vi "メイン.vi"() -> (2 "測定周期/ms":dbl, 3 "値転記用配列":T2[](array[typedef]))   [LabVIEW 2021] (continued)
        n4326 = for {
          N: w6937 -> [_]
          tunnel: FALSE -> [w6949]
          i -> [w6950]
          n4327 = case shown="5" w6950 {
            tunnel: w6949 -> [w6951 w6952 w6953 w6954 w6955 _ w6956 w6957 w6958 w6959 w6960 w6961]
            frame 0, Default {
              n4328 = local write "測定新値\nリセット用 1"(w6951) -> ()
            }
            frame 1 {
              n4329 = local write "測定新値\nリセット用 2"(w6952) -> ()
            }
            frame 2 {
              n4330 = local write "測定新値\nリセット用 3"(w6953) -> ()
            }
            frame 3 {
              n4331 = local write "測定新値\nリセット用 4"(w6954) -> ()
            }
            frame 4 {
              n4332 = local write "測定新値\nリセット用 5"(w6955) -> ()
            }
            frame 5 {
            }
            frame 6 {
              n4333 = local write "測定新値\nリセット用 7"(w6956) -> ()
            }
            frame 7 {
              n4334 = local write "測定新値\nリセット用 8"(w6957) -> ()
            }
            frame 8 {
              n4335 = local write "測定新値\nリセット用 9"(w6958) -> ()
            }
            frame 9 {
              n4336 = local write "測定新値\nリセット用 10"(w6959) -> ()
            }
            frame 10 {
              n4337 = local write "測定新値\nリセット用 11"(w6960) -> ()
            }
            frame 11 {
              n4338 = local write "測定新値\nリセット用 12"(w6961) -> ()
            }
          }
        }
        n4339 = for {
          N: w6937 -> [_]
          tunnel: w6943 -> [w6962]
          i -> [w6963]
          n4340 = case shown="11" w6963 {
            tunnel: w6962 -> [w6964 w6965 w6966 w6967 w6968 w6969 w6970 w6971 w6972 w6973 w6974 w6975]
            frame 0, Default {
              n4341 = property on="メイン測定ボタン_単発 1" class="Bool (指定)"("DisabledEnum"=w6964) -> ()  [unwired: 2 in, 2 out]
              n4342 = property on="メイン測定ボタン_連続 1" class="Bool (指定)"("DisabledEnum"=w6964) -> ()  [unwired: 2 in, 2 out]
            }
            frame 1 {
              n4343 = property on="メイン測定ボタン_単発 2" class="Bool (指定)"("DisabledEnum"=w6965) -> ()  [unwired: 2 in, 2 out]
              n4344 = property on="メイン測定ボタン_連続 2" class="Bool (指定)"("DisabledEnum"=w6965) -> ()  [unwired: 2 in, 2 out]
            }
            frame 2 {
              n4345 = property on="メイン測定ボタン_単発 3" class="Bool (指定)"("DisabledEnum"=w6966) -> ()  [unwired: 2 in, 2 out]
              n4346 = property on="メイン測定ボタン_連続 3" class="Bool (指定)"("DisabledEnum"=w6966) -> ()  [unwired: 2 in, 2 out]
            }
            frame 3 {
              n4347 = property on="メイン測定ボタン_単発 4" class="Bool (指定)"("DisabledEnum"=w6967) -> ()  [unwired: 2 in, 2 out]
              n4348 = property on="メイン測定ボタン_連続 4" class="Bool (指定)"("DisabledEnum"=w6967) -> ()  [unwired: 2 in, 2 out]
            }
            frame 4 {
              n4349 = property on="メイン測定ボタン_単発 5" class="Bool (指定)"("DisabledEnum"=w6968) -> ()  [unwired: 2 in, 2 out]
              n4350 = property on="メイン測定ボタン_連続 5" class="Bool (指定)"("DisabledEnum"=w6968) -> ()  [unwired: 2 in, 2 out]
            }
            frame 5 {
              n4351 = property on="メイン測定ボタン_単発 6" class="Bool (指定)"("DisabledEnum"=w6969) -> ()  [unwired: 2 in, 2 out]
            }
            frame 6 {
              n4352 = property on="メイン測定ボタン_連続 7" class="Bool (指定)"("DisabledEnum"=w6970) -> ()  [unwired: 2 in, 2 out]
              n4353 = property on="メイン測定ボタン_単発 7" class="Bool (指定)"("DisabledEnum"=w6970) -> ()  [unwired: 2 in, 2 out]
            }
            frame 7 {
              n4354 = property on="メイン測定ボタン_単発 8" class="Bool (指定)"("DisabledEnum"=w6971) -> ()  [unwired: 2 in, 2 out]
              n4355 = property on="メイン測定ボタン_連続 8" class="Bool (指定)"("DisabledEnum"=w6971) -> ()  [unwired: 2 in, 2 out]
            }
            frame 8 {
              n4356 = property on="メイン測定ボタン_単発 9" class="Bool (指定)"("DisabledEnum"=w6972) -> ()  [unwired: 2 in, 2 out]
              n4357 = property on="メイン測定ボタン_連続 9" class="Bool (指定)"("DisabledEnum"=w6972) -> ()  [unwired: 2 in, 2 out]
            }
            frame 9 {
              n4358 = property on="メイン測定ボタン_単発 10" class="Bool (指定)"("DisabledEnum"=w6973) -> ()  [unwired: 2 in, 2 out]
              n4359 = property on="メイン測定ボタン_連続 10" class="Bool (指定)"("DisabledEnum"=w6973) -> ()  [unwired: 2 in, 2 out]
            }
            frame 10 {
              n4360 = property on="メイン測定ボタン_単発 11" class="Bool (指定)"("DisabledEnum"=w6974) -> ()  [unwired: 2 in, 2 out]
              n4361 = property on="メイン測定ボタン_連続 11" class="Bool (指定)"("DisabledEnum"=w6974) -> ()  [unwired: 2 in, 2 out]
            }
            frame 11 {
              n4362 = property on="メイン測定ボタン_連続 12" class="Bool (指定)"("DisabledEnum"=w6975) -> ()  [unwired: 2 in, 2 out]
              n4363 = property on="メイン測定ボタン_単発 12" class="Bool (指定)"("DisabledEnum"=w6975) -> ()  [unwired: 2 in, 2 out]
            }
          }
        }
        n4364 = property on="TOPページへ" class="Bool"("DisabledEnum"=w6943) -> ()  [unwired: 2 in, 2 out]
        n4365 = property on="保存して終了" class="Bool"("DisabledEnum"=w6943) -> ()  [unwired: 2 in, 2 out]
        n4366 = property on="保存せずに" class="Bool"("DisabledEnum"=w6943) -> ()  [unwired: 2 in, 2 out]
      }
      event Value Change {
        w6976 = 12
        # "④ボタン操作時の他のボタン操作無効"
        # "※複製時\n①ブールボタン\n測定旧値\nが複製されているか確認\n②測定新値リセット用の作成\n対象の以外をリセットする\n③\nキュー\n④対象の連続ボタン以外複製する"
        # "③"
        # "旧値(ボタンが押される前と後)の値でグローバル_測定キャンセルボタンの\nTrue/Falseの切り替えを行う"
        # "②　例ケースが”メイン測定ボタン_連続2”の場合、\n測定新値リセット用2以外をリセットする"
        # "①"
        n4367 = event-data() -> ("OldVal"=w6978:T6)  [unwired: 1 in, 2 out]
        "測定旧値 7" <- w6978
        n4368 = Enqueue Element(queue=w6986, element="測定7", error in (no error)=w6983) -> (queue out=w6985:refnum<queue>, error out=w6984:errorcluster)  [unwired: 1 in, 1 out]
        n4369 = Select(t=TRUE, s=w6978, f=FALSE) -> (s? t:f=w6981:bool)
        n4370 = global write "測定キャンセルボタン.vi" "グローバル_測定キャンセルボタン"(w6981) -> ()
        n4371 = local write "G_メイン測定キャンセルボタン"(w6981) -> ()
        n4372 = for {
          N: w6976 -> [_]
          tunnel: FALSE -> [w6988]
          i -> [w6989]
          n4373 = case shown="6" w6989 {
            tunnel: w6988 -> [w6990 w6991 w6992 w6993 w6994 w6995 _ w6996 w6997 w6998 w6999 w7000]
            frame 0, Default {
              n4374 = local write "測定新値\nリセット用 1"(w6990) -> ()
            }
            frame 1 {
              n4375 = local write "測定新値\nリセット用 2"(w6991) -> ()
            }
            frame 2 {
              n4376 = local write "測定新値\nリセット用 3"(w6992) -> ()
            }
            frame 3 {
              n4377 = local write "測定新値\nリセット用 4"(w6993) -> ()
            }
            frame 4 {
              n4378 = local write "測定新値\nリセット用 5"(w6994) -> ()
            }
            frame 5 {
              n4379 = local write "測定新値\nリセット用 6"(w6995) -> ()
            }
            frame 6 {
            }
            frame 7 {
              n4380 = local write "測定新値\nリセット用 8"(w6996) -> ()
            }
            frame 8 {
              n4381 = local write "測定新値\nリセット用 9"(w6997) -> ()
            }
            frame 9 {
              n4382 = local write "測定新値\nリセット用 10"(w6998) -> ()
            }
            frame 10 {
              n4383 = local write "測定新値\nリセット用 11"(w6999) -> ()
            }
            frame 11 {
              n4384 = local write "測定新値\nリセット用 12"(w7000) -> ()
            }
          }
        }
        n4385 = for {
          N: w6976 -> [_]
          tunnel: w6982 -> [w7001]
          i -> [w7002]
          n4386 = case shown="11" w7002 {
            tunnel: w7001 -> [w7003 w7004 w7005 w7006 w7007 w7008 w7009 w7010 w7011 w7012 w7013 w7014]
            frame 0, Default {
              n4387 = property on="メイン測定ボタン_単発 1" class="Bool (指定)"("DisabledEnum"=w7003) -> ()  [unwired: 2 in, 2 out]
              n4388 = property on="メイン測定ボタン_連続 1" class="Bool (指定)"("DisabledEnum"=w7003) -> ()  [unwired: 2 in, 2 out]
            }
            frame 1 {
              n4389 = property on="メイン測定ボタン_単発 2" class="Bool (指定)"("DisabledEnum"=w7004) -> ()  [unwired: 2 in, 2 out]
              n4390 = property on="メイン測定ボタン_連続 2" class="Bool (指定)"("DisabledEnum"=w7004) -> ()  [unwired: 2 in, 2 out]
            }
            frame 2 {
              n4391 = property on="メイン測定ボタン_単発 3" class="Bool (指定)"("DisabledEnum"=w7005) -> ()  [unwired: 2 in, 2 out]
              n4392 = property on="メイン測定ボタン_連続 3" class="Bool (指定)"("DisabledEnum"=w7005) -> ()  [unwired: 2 in, 2 out]
            }
            frame 3 {
              n4393 = property on="メイン測定ボタン_単発 4" class="Bool (指定)"("DisabledEnum"=w7006) -> ()  [unwired: 2 in, 2 out]
              n4394 = property on="メイン測定ボタン_連続 4" class="Bool (指定)"("DisabledEnum"=w7006) -> ()  [unwired: 2 in, 2 out]
            }
            frame 4 {
              n4395 = property on="メイン測定ボタン_単発 5" class="Bool (指定)"("DisabledEnum"=w7007) -> ()  [unwired: 2 in, 2 out]
              n4396 = property on="メイン測定ボタン_連続 5" class="Bool (指定)"("DisabledEnum"=w7007) -> ()  [unwired: 2 in, 2 out]
            }
            frame 5 {
              n4397 = property on="メイン測定ボタン_連続 6" class="Bool (指定)"("DisabledEnum"=w7008) -> ()  [unwired: 2 in, 2 out]
              n4398 = property on="メイン測定ボタン_単発 6" class="Bool (指定)"("DisabledEnum"=w7008) -> ()  [unwired: 2 in, 2 out]
            }
            frame 6 {
              n4399 = property on="メイン測定ボタン_単発 7" class="Bool (指定)"("DisabledEnum"=w7009) -> ()  [unwired: 2 in, 2 out]
            }
            frame 7 {
              n4400 = property on="メイン測定ボタン_単発 8" class="Bool (指定)"("DisabledEnum"=w7010) -> ()  [unwired: 2 in, 2 out]
              n4401 = property on="メイン測定ボタン_連続 8" class="Bool (指定)"("DisabledEnum"=w7010) -> ()  [unwired: 2 in, 2 out]
            }
            frame 8 {
              n4402 = property on="メイン測定ボタン_単発 9" class="Bool (指定)"("DisabledEnum"=w7011) -> ()  [unwired: 2 in, 2 out]
              n4403 = property on="メイン測定ボタン_連続 9" class="Bool (指定)"("DisabledEnum"=w7011) -> ()  [unwired: 2 in, 2 out]
            }
            frame 9 {
              n4404 = property on="メイン測定ボタン_単発 10" class="Bool (指定)"("DisabledEnum"=w7012) -> ()  [unwired: 2 in, 2 out]
              n4405 = property on="メイン測定ボタン_連続 10" class="Bool (指定)"("DisabledEnum"=w7012) -> ()  [unwired: 2 in, 2 out]
            }
            frame 10 {
              n4406 = property on="メイン測定ボタン_単発 11" class="Bool (指定)"("DisabledEnum"=w7013) -> ()  [unwired: 2 in, 2 out]
              n4407 = property on="メイン測定ボタン_連続 11" class="Bool (指定)"("DisabledEnum"=w7013) -> ()  [unwired: 2 in, 2 out]
            }
            frame 11 {
              n4408 = property on="メイン測定ボタン_連続 12" class="Bool (指定)"("DisabledEnum"=w7014) -> ()  [unwired: 2 in, 2 out]
              n4409 = property on="メイン測定ボタン_単発 12" class="Bool (指定)"("DisabledEnum"=w7014) -> ()  [unwired: 2 in, 2 out]
            }
          }
        }
        n4410 = property on="TOPページへ" class="Bool"("DisabledEnum"=w6982) -> ()  [unwired: 2 in, 2 out]
        n4411 = property on="保存して終了" class="Bool"("DisabledEnum"=w6982) -> ()  [unwired: 2 in, 2 out]
        n4412 = property on="保存せずに" class="Bool"("DisabledEnum"=w6982) -> ()  [unwired: 2 in, 2 out]
      }
      event Value Change {
        w7015 = 12
        # "④ボタン操作時の他のボタン操作無効"
        # "※複製時\n①ブールボタン\n測定旧値\nが複製されているか確認\n②測定新値リセット用の作成\n対象の以外をリセットする\n③\nキュー\n④対象の連続ボタン以外複製する"
        # "③"
        # "旧値(ボタンが押される前と後)の値でグローバル_測定キャンセルボタンの\nTrue/Falseの切り替えを行う"
        # "②　例ケースが”メイン測定ボタン_連続2”の場合、\n測定新値リセット用2以外をリセットする"
        # "①"
        n4413 = event-data() -> ("OldVal"=w7017:T6)  [unwired: 1 in, 2 out]
        "測定旧値 8" <- w7017
        n4414 = Enqueue Element(queue=w7025, element="測定8", error in (no error)=w7022) -> (queue out=w7024:refnum<queue>, error out=w7023:errorcluster)  [unwired: 1 in, 1 out]
        n4415 = Select(t=TRUE, s=w7017, f=FALSE) -> (s? t:f=w7020:bool)
        n4416 = global write "測定キャンセルボタン.vi" "グローバル_測定キャンセルボタン"(w7020) -> ()
        n4417 = local write "G_メイン測定キャンセルボタン"(w7020) -> ()
        n4418 = for {
          N: w7015 -> [_]
          tunnel: FALSE -> [w7027]
          i -> [w7028]
          n4419 = case shown="7" w7028 {
            tunnel: w7027 -> [w7029 w7030 w7031 w7032 w7033 w7034 w7035 _ w7036 w7037 w7038 w7039]
            frame 0, Default {
              n4420 = local write "測定新値\nリセット用 1"(w7029) -> ()
            }
            frame 1 {
              n4421 = local write "測定新値\nリセット用 2"(w7030) -> ()
            }
            frame 2 {
              n4422 = local write "測定新値\nリセット用 3"(w7031) -> ()
            }
            frame 3 {
              n4423 = local write "測定新値\nリセット用 4"(w7032) -> ()
            }
            frame 4 {
              n4424 = local write "測定新値\nリセット用 5"(w7033) -> ()
            }
            frame 5 {
              n4425 = local write "測定新値\nリセット用 6"(w7034) -> ()
            }
            frame 6 {
              n4426 = local write "測定新値\nリセット用 7"(w7035) -> ()
            }
            frame 7 {
            }
            frame 8 {
              n4427 = local write "測定新値\nリセット用 9"(w7036) -> ()
            }
            frame 9 {
              n4428 = local write "測定新値\nリセット用 10"(w7037) -> ()
            }
            frame 10 {
              n4429 = local write "測定新値\nリセット用 11"(w7038) -> ()
            }
            frame 11 {
              n4430 = local write "測定新値\nリセット用 12"(w7039) -> ()
            }
          }
        }
        n4431 = for {
          N: w7015 -> [_]
          tunnel: w7021 -> [w7040]
          i -> [w7041]
          n4432 = case shown="11" w7041 {
            tunnel: w7040 -> [w7042 w7043 w7044 w7045 w7046 w7047 w7048 w7049 w7050 w7051 w7052 w7053]
            frame 0, Default {
              n4433 = property on="メイン測定ボタン_単発 1" class="Bool (指定)"("DisabledEnum"=w7042) -> ()  [unwired: 2 in, 2 out]
              n4434 = property on="メイン測定ボタン_連続 1" class="Bool (指定)"("DisabledEnum"=w7042) -> ()  [unwired: 2 in, 2 out]
            }
            frame 1 {
              n4435 = property on="メイン測定ボタン_単発 2" class="Bool (指定)"("DisabledEnum"=w7043) -> ()  [unwired: 2 in, 2 out]
              n4436 = property on="メイン測定ボタン_連続 2" class="Bool (指定)"("DisabledEnum"=w7043) -> ()  [unwired: 2 in, 2 out]
            }
            frame 2 {
              n4437 = property on="メイン測定ボタン_単発 3" class="Bool (指定)"("DisabledEnum"=w7044) -> ()  [unwired: 2 in, 2 out]
              n4438 = property on="メイン測定ボタン_連続 3" class="Bool (指定)"("DisabledEnum"=w7044) -> ()  [unwired: 2 in, 2 out]
            }
            frame 3 {
              n4439 = property on="メイン測定ボタン_単発 4" class="Bool (指定)"("DisabledEnum"=w7045) -> ()  [unwired: 2 in, 2 out]
              n4440 = property on="メイン測定ボタン_連続 4" class="Bool (指定)"("DisabledEnum"=w7045) -> ()  [unwired: 2 in, 2 out]
            }
            frame 4 {
              n4441 = property on="メイン測定ボタン_単発 5" class="Bool (指定)"("DisabledEnum"=w7046) -> ()  [unwired: 2 in, 2 out]
              n4442 = property on="メイン測定ボタン_連続 5" class="Bool (指定)"("DisabledEnum"=w7046) -> ()  [unwired: 2 in, 2 out]
            }
            frame 5 {
              n4443 = property on="メイン測定ボタン_連続 6" class="Bool (指定)"("DisabledEnum"=w7047) -> ()  [unwired: 2 in, 2 out]
              n4444 = property on="メイン測定ボタン_単発 6" class="Bool (指定)"("DisabledEnum"=w7047) -> ()  [unwired: 2 in, 2 out]
            }
            frame 6 {
              n4445 = property on="メイン測定ボタン_連続 7" class="Bool (指定)"("DisabledEnum"=w7048) -> ()  [unwired: 2 in, 2 out]
              n4446 = property on="メイン測定ボタン_単発 7" class="Bool (指定)"("DisabledEnum"=w7048) -> ()  [unwired: 2 in, 2 out]
            }
            frame 7 {
              n4447 = property on="メイン測定ボタン_単発 8" class="Bool (指定)"("DisabledEnum"=w7049) -> ()  [unwired: 2 in, 2 out]
            }
            frame 8 {
              n4448 = property on="メイン測定ボタン_単発 9" class="Bool (指定)"("DisabledEnum"=w7050) -> ()  [unwired: 2 in, 2 out]
              n4449 = property on="メイン測定ボタン_連続 9" class="Bool (指定)"("DisabledEnum"=w7050) -> ()  [unwired: 2 in, 2 out]
            }
            frame 9 {
              n4450 = property on="メイン測定ボタン_単発 10" class="Bool (指定)"("DisabledEnum"=w7051) -> ()  [unwired: 2 in, 2 out]
              n4451 = property on="メイン測定ボタン_連続 10" class="Bool (指定)"("DisabledEnum"=w7051) -> ()  [unwired: 2 in, 2 out]
            }
            frame 10 {
              n4452 = property on="メイン測定ボタン_単発 11" class="Bool (指定)"("DisabledEnum"=w7052) -> ()  [unwired: 2 in, 2 out]
              n4453 = property on="メイン測定ボタン_連続 11" class="Bool (指定)"("DisabledEnum"=w7052) -> ()  [unwired: 2 in, 2 out]
            }
            frame 11 {
              n4454 = property on="メイン測定ボタン_連続 12" class="Bool (指定)"("DisabledEnum"=w7053) -> ()  [unwired: 2 in, 2 out]
              n4455 = property on="メイン測定ボタン_単発 12" class="Bool (指定)"("DisabledEnum"=w7053) -> ()  [unwired: 2 in, 2 out]
            }
          }
        }
        n4456 = property on="TOPページへ" class="Bool"("DisabledEnum"=w7021) -> ()  [unwired: 2 in, 2 out]
        n4457 = property on="保存して終了" class="Bool"("DisabledEnum"=w7021) -> ()  [unwired: 2 in, 2 out]
        n4458 = property on="保存せずに" class="Bool"("DisabledEnum"=w7021) -> ()  [unwired: 2 in, 2 out]
      }
      event Value Change {
        w7054 = 12
        # "④ボタン操作時の他のボタン操作無効"
        # "※複製時\n①ブールボタン\n測定旧値\nが複製されているか確認\n②測定新値リセット用の作成\n対象の以外をリセットする\n③\nキュー\n④対象の連続ボタン以外複製する"
        # "③"
        # "旧値(ボタンが押される前と後)の値でグローバル_測定キャンセルボタンの\nTrue/Falseの切り替えを行う"
        # "②　例ケースが”メイン測定ボタン_連続2”の場合、\n測定新値リセット用2以外をリセットする"
        # "①"
        n4459 = event-data() -> ("OldVal"=w7056:T6)  [unwired: 1 in, 2 out]
        "測定旧値 9" <- w7056
        n4460 = Enqueue Element(queue=w7064, element="測定9", error in (no error)=w7061) -> (queue out=w7063:refnum<queue>, error out=w7062:errorcluster)  [unwired: 1 in, 1 out]
        n4461 = Select(t=TRUE, s=w7056, f=FALSE) -> (s? t:f=w7059:bool)
        n4462 = global write "測定キャンセルボタン.vi" "グローバル_測定キャンセルボタン"(w7059) -> ()
        n4463 = local write "G_メイン測定キャンセルボタン"(w7059) -> ()
        n4464 = for {
          N: w7054 -> [_]
          tunnel: FALSE -> [w7066]
          i -> [w7067]
          n4465 = case shown="8" w7067 {
            tunnel: w7066 -> [w7068 w7069 w7070 w7071 w7072 w7073 w7074 w7075 _ w7076 w7077 w7078]
            frame 0, Default {
              n4466 = local write "測定新値\nリセット用 1"(w7068) -> ()
            }
            frame 1 {
              n4467 = local write "測定新値\nリセット用 2"(w7069) -> ()
            }
            frame 2 {
              n4468 = local write "測定新値\nリセット用 3"(w7070) -> ()
            }
            frame 3 {
              n4469 = local write "測定新値\nリセット用 4"(w7071) -> ()
            }
            frame 4 {
              n4470 = local write "測定新値\nリセット用 5"(w7072) -> ()
            }
            frame 5 {
              n4471 = local write "測定新値\nリセット用 6"(w7073) -> ()
            }
            frame 6 {
              n4472 = local write "測定新値\nリセット用 7"(w7074) -> ()
            }
            frame 7 {
              n4473 = local write "測定新値\nリセット用 8"(w7075) -> ()
            }
            frame 8 {
            }
            frame 9 {
              n4474 = local write "測定新値\nリセット用 10"(w7076) -> ()
            }
            frame 10 {
              n4475 = local write "測定新値\nリセット用 11"(w7077) -> ()
            }
            frame 11 {
              n4476 = local write "測定新値\nリセット用 12"(w7078) -> ()
            }
          }
        }
        n4477 = for {
          N: w7054 -> [_]
          tunnel: w7060 -> [w7079]
          i -> [w7080]
          n4478 = case shown="11" w7080 {
            tunnel: w7079 -> [w7081 w7082 w7083 w7084 w7085 w7086 w7087 w7088 w7089 w7090 w7091 w7092]
            frame 0, Default {
              n4479 = property on="メイン測定ボタン_単発 1" class="Bool (指定)"("DisabledEnum"=w7081) -> ()  [unwired: 2 in, 2 out]
              n4480 = property on="メイン測定ボタン_連続 1" class="Bool (指定)"("DisabledEnum"=w7081) -> ()  [unwired: 2 in, 2 out]
            }
            frame 1 {
              n4481 = property on="メイン測定ボタン_単発 2" class="Bool (指定)"("DisabledEnum"=w7082) -> ()  [unwired: 2 in, 2 out]
              n4482 = property on="メイン測定ボタン_連続 2" class="Bool (指定)"("DisabledEnum"=w7082) -> ()  [unwired: 2 in, 2 out]
            }
            frame 2 {
              n4483 = property on="メイン測定ボタン_単発 3" class="Bool (指定)"("DisabledEnum"=w7083) -> ()  [unwired: 2 in, 2 out]
              n4484 = property on="メイン測定ボタン_連続 3" class="Bool (指定)"("DisabledEnum"=w7083) -> ()  [unwired: 2 in, 2 out]
            }
            frame 3 {
              n4485 = property on="メイン測定ボタン_単発 4" class="Bool (指定)"("DisabledEnum"=w7084) -> ()  [unwired: 2 in, 2 out]
              n4486 = property on="メイン測定ボタン_連続 4" class="Bool (指定)"("DisabledEnum"=w7084) -> ()  [unwired: 2 in, 2 out]
            }
            frame 4 {
              n4487 = property on="メイン測定ボタン_単発 5" class="Bool (指定)"("DisabledEnum"=w7085) -> ()  [unwired: 2 in, 2 out]
              n4488 = property on="メイン測定ボタン_連続 5" class="Bool (指定)"("DisabledEnum"=w7085) -> ()  [unwired: 2 in, 2 out]
            }
            frame 5 {
              n4489 = property on="メイン測定ボタン_連続 6" class="Bool (指定)"("DisabledEnum"=w7086) -> ()  [unwired: 2 in, 2 out]
              n4490 = property on="メイン測定ボタン_単発 6" class="Bool (指定)"("DisabledEnum"=w7086) -> ()  [unwired: 2 in, 2 out]
            }
            frame 6 {
              n4491 = property on="メイン測定ボタン_連続 7" class="Bool (指定)"("DisabledEnum"=w7087) -> ()  [unwired: 2 in, 2 out]
              n4492 = property on="メイン測定ボタン_単発 7" class="Bool (指定)"("DisabledEnum"=w7087) -> ()  [unwired: 2 in, 2 out]
            }
            frame 7 {
              n4493 = property on="メイン測定ボタン_単発 8" class="Bool (指定)"("DisabledEnum"=w7088) -> ()  [unwired: 2 in, 2 out]
              n4494 = property on="メイン測定ボタン_連続 8" class="Bool (指定)"("DisabledEnum"=w7088) -> ()  [unwired: 2 in, 2 out]
            }
            frame 8 {
              n4495 = property on="メイン測定ボタン_単発 9" class="Bool (指定)"("DisabledEnum"=w7089) -> ()  [unwired: 2 in, 2 out]
            }
            frame 9 {
              n4496 = property on="メイン測定ボタン_単発 10" class="Bool (指定)"("DisabledEnum"=w7090) -> ()  [unwired: 2 in, 2 out]
              n4497 = property on="メイン測定ボタン_連続 10" class="Bool (指定)"("DisabledEnum"=w7090) -> ()  [unwired: 2 in, 2 out]
            }
            frame 10 {
              n4498 = property on="メイン測定ボタン_単発 11" class="Bool (指定)"("DisabledEnum"=w7091) -> ()  [unwired: 2 in, 2 out]
              n4499 = property on="メイン測定ボタン_連続 11" class="Bool (指定)"("DisabledEnum"=w7091) -> ()  [unwired: 2 in, 2 out]
            }
            frame 11 {
              n4500 = property on="メイン測定ボタン_連続 12" class="Bool (指定)"("DisabledEnum"=w7092) -> ()  [unwired: 2 in, 2 out]
              n4501 = property on="メイン測定ボタン_単発 12" class="Bool (指定)"("DisabledEnum"=w7092) -> ()  [unwired: 2 in, 2 out]
            }
          }
        }
        n4502 = property on="TOPページへ" class="Bool"("DisabledEnum"=w7060) -> ()  [unwired: 2 in, 2 out]
        n4503 = property on="保存して終了" class="Bool"("DisabledEnum"=w7060) -> ()  [unwired: 2 in, 2 out]
        n4504 = property on="保存せずに" class="Bool"("DisabledEnum"=w7060) -> ()  [unwired: 2 in, 2 out]
      }
      event Value Change {
        w7093 = 12
        # "④ボタン操作時の他のボタン操作無効"
        # "※複製時\n①ブールボタン\n測定旧値\nが複製されているか確認\n②測定新値リセット用の作成\n対象の以外をリセットする\n③\nキュー\n④対象の連続ボタン以外複製する"
        # "③"
        # "旧値(ボタンが押される前と後)の値でグローバル_測定キャンセルボタンの\nTrue/Falseの切り替えを行う"
        # "②　例ケースが”メイン測定ボタン_連続2”の場合、\n測定新値リセット用2以外をリセットする"
        # "①"
        n4505 = event-data() -> ("OldVal"=w7095:T6)  [unwired: 1 in, 2 out]
        "測定旧値 10" <- w7095
        n4506 = Enqueue Element(queue=w7103, element="測定10", error in (no error)=w7100) -> (queue out=w7102:refnum<queue>, error out=w7101:errorcluster)  [unwired: 1 in, 1 out]
        n4507 = Select(t=TRUE, s=w7095, f=FALSE) -> (s? t:f=w7098:bool)
        n4508 = global write "測定キャンセルボタン.vi" "グローバル_測定キャンセルボタン"(w7098) -> ()
        n4509 = local write "G_メイン測定キャンセルボタン"(w7098) -> ()
        n4510 = for {
          N: w7093 -> [_]
          tunnel: FALSE -> [w7105]
          i -> [w7106]
          n4511 = case shown="9" w7106 {
            tunnel: w7105 -> [w7107 w7108 w7109 w7110 w7111 w7112 w7113 w7114 w7115 _ w7116 w7117]
            frame 0, Default {
              n4512 = local write "測定新値\nリセット用 1"(w7107) -> ()
            }
            frame 1 {
              n4513 = local write "測定新値\nリセット用 2"(w7108) -> ()
            }
            frame 2 {
              n4514 = local write "測定新値\nリセット用 3"(w7109) -> ()
            }
            frame 3 {
              n4515 = local write "測定新値\nリセット用 4"(w7110) -> ()
            }
            frame 4 {
              n4516 = local write "測定新値\nリセット用 5"(w7111) -> ()
            }
            frame 5 {
              n4517 = local write "測定新値\nリセット用 6"(w7112) -> ()
            }
            frame 6 {
              n4518 = local write "測定新値\nリセット用 7"(w7113) -> ()
            }
            frame 7 {
              n4519 = local write "測定新値\nリセット用 8"(w7114) -> ()
            }
            frame 8 {
              n4520 = local write "測定新値\nリセット用 9"(w7115) -> ()
            }
            frame 9 {
            }
            frame 10 {
              n4521 = local write "測定新値\nリセット用 11"(w7116) -> ()
            }
            frame 11 {
              n4522 = local write "測定新値\nリセット用 12"(w7117) -> ()
            }
          }
        }
        n4523 = for {
          N: w7093 -> [_]
          tunnel: w7099 -> [w7118]
          i -> [w7119]
          n4524 = case shown="11" w7119 {
            tunnel: w7118 -> [w7120 w7121 w7122 w7123 w7124 w7125 w7126 w7127 w7128 w7129 w7130 w7131]
            frame 0, Default {
              n4525 = property on="メイン測定ボタン_単発 1" class="Bool (指定)"("DisabledEnum"=w7120) -> ()  [unwired: 2 in, 2 out]
              n4526 = property on="メイン測定ボタン_連続 1" class="Bool (指定)"("DisabledEnum"=w7120) -> ()  [unwired: 2 in, 2 out]
            }
            frame 1 {
              n4527 = property on="メイン測定ボタン_単発 2" class="Bool (指定)"("DisabledEnum"=w7121) -> ()  [unwired: 2 in, 2 out]
              n4528 = property on="メイン測定ボタン_連続 2" class="Bool (指定)"("DisabledEnum"=w7121) -> ()  [unwired: 2 in, 2 out]
            }
            frame 2 {
              n4529 = property on="メイン測定ボタン_単発 3" class="Bool (指定)"("DisabledEnum"=w7122) -> ()  [unwired: 2 in, 2 out]
              n4530 = property on="メイン測定ボタン_連続 3" class="Bool (指定)"("DisabledEnum"=w7122) -> ()  [unwired: 2 in, 2 out]
            }
            frame 3 {
              n4531 = property on="メイン測定ボタン_単発 4" class="Bool (指定)"("DisabledEnum"=w7123) -> ()  [unwired: 2 in, 2 out]
              n4532 = property on="メイン測定ボタン_連続 4" class="Bool (指定)"("DisabledEnum"=w7123) -> ()  [unwired: 2 in, 2 out]
            }
            frame 4 {
              n4533 = property on="メイン測定ボタン_単発 5" class="Bool (指定)"("DisabledEnum"=w7124) -> ()  [unwired: 2 in, 2 out]
              n4534 = property on="メイン測定ボタン_連続 5" class="Bool (指定)"("DisabledEnum"=w7124) -> ()  [unwired: 2 in, 2 out]
            }
            frame 5 {
              n4535 = property on="メイン測定ボタン_連続 6" class="Bool (指定)"("DisabledEnum"=w7125) -> ()  [unwired: 2 in, 2 out]
              n4536 = property on="メイン測定ボタン_単発 6" class="Bool (指定)"("DisabledEnum"=w7125) -> ()  [unwired: 2 in, 2 out]
            }
            frame 6 {
              n4537 = property on="メイン測定ボタン_連続 7" class="Bool (指定)"("DisabledEnum"=w7126) -> ()  [unwired: 2 in, 2 out]
              n4538 = property on="メイン測定ボタン_単発 7" class="Bool (指定)"("DisabledEnum"=w7126) -> ()  [unwired: 2 in, 2 out]
            }
            frame 7 {
              n4539 = property on="メイン測定ボタン_単発 8" class="Bool (指定)"("DisabledEnum"=w7127) -> ()  [unwired: 2 in, 2 out]
              n4540 = property on="メイン測定ボタン_連続 8" class="Bool (指定)"("DisabledEnum"=w7127) -> ()  [unwired: 2 in, 2 out]
            }
            frame 8 {
              n4541 = property on="メイン測定ボタン_単発 9" class="Bool (指定)"("DisabledEnum"=w7128) -> ()  [unwired: 2 in, 2 out]
              n4542 = property on="メイン測定ボタン_連続 9" class="Bool (指定)"("DisabledEnum"=w7128) -> ()  [unwired: 2 in, 2 out]
            }
            frame 9 {
              n4543 = property on="メイン測定ボタン_単発 10" class="Bool (指定)"("DisabledEnum"=w7129) -> ()  [unwired: 2 in, 2 out]
            }
            frame 10 {
              n4544 = property on="メイン測定ボタン_単発 11" class="Bool (指定)"("DisabledEnum"=w7130) -> ()  [unwired: 2 in, 2 out]
              n4545 = property on="メイン測定ボタン_連続 11" class="Bool (指定)"("DisabledEnum"=w7130) -> ()  [unwired: 2 in, 2 out]
            }
            frame 11 {
              n4546 = property on="メイン測定ボタン_連続 12" class="Bool (指定)"("DisabledEnum"=w7131) -> ()  [unwired: 2 in, 2 out]
              n4547 = property on="メイン測定ボタン_単発 12" class="Bool (指定)"("DisabledEnum"=w7131) -> ()  [unwired: 2 in, 2 out]
            }
          }
        }
        n4548 = property on="TOPページへ" class="Bool"("DisabledEnum"=w7099) -> ()  [unwired: 2 in, 2 out]
        n4549 = property on="保存して終了" class="Bool"("DisabledEnum"=w7099) -> ()  [unwired: 2 in, 2 out]
        n4550 = property on="保存せずに" class="Bool"("DisabledEnum"=w7099) -> ()  [unwired: 2 in, 2 out]
      }
      event Value Change {
        w7132 = 12
        # "④ボタン操作時の他のボタン操作無効"
        # "※複製時\n①ブールボタン\n測定旧値\nが複製されているか確認\n②測定新値リセット用の作成\n対象の以外をリセットする\n③\nキュー\n④対象の連続ボタン以外複製する"
        # "③"
        # "旧値(ボタンが押される前と後)の値でグローバル_測定キャンセルボタンの\nTrue/Falseの切り替えを行う"
        # "②　例ケースが”メイン測定ボタン_連続2”の場合、\n測定新値リセット用2以外をリセットする"
        # "①"
        n4551 = event-data() -> ("OldVal"=w7134:T6)  [unwired: 1 in, 2 out]
        "測定旧値 11" <- w7134
        n4552 = Enqueue Element(queue=w7142, element="測定11", error in (no error)=w7139) -> (queue out=w7141:refnum<queue>, error out=w7140:errorcluster)  [unwired: 1 in, 1 out]
        n4553 = Select(t=TRUE, s=w7134, f=FALSE) -> (s? t:f=w7137:bool)
        n4554 = global write "測定キャンセルボタン.vi" "グローバル_測定キャンセルボタン"(w7137) -> ()
        n4555 = local write "G_メイン測定キャンセルボタン"(w7137) -> ()
        n4556 = for {
          N: w7132 -> [_]
          tunnel: FALSE -> [w7144]
          i -> [w7145]
          n4557 = case shown="10" w7145 {
            tunnel: w7144 -> [w7146 w7147 w7148 w7149 w7150 w7151 w7152 w7153 w7154 w7155 _ w7156]
            frame 0, Default {
              n4558 = local write "測定新値\nリセット用 1"(w7146) -> ()
            }
            frame 1 {
              n4559 = local write "測定新値\nリセット用 2"(w7147) -> ()
            }
            frame 2 {
              n4560 = local write "測定新値\nリセット用 3"(w7148) -> ()
            }
            frame 3 {
              n4561 = local write "測定新値\nリセット用 4"(w7149) -> ()
            }
            frame 4 {
              n4562 = local write "測定新値\nリセット用 5"(w7150) -> ()
            }
            frame 5 {
              n4563 = local write "測定新値\nリセット用 6"(w7151) -> ()
            }
            frame 6 {
              n4564 = local write "測定新値\nリセット用 7"(w7152) -> ()
            }
            frame 7 {
              n4565 = local write "測定新値\nリセット用 8"(w7153) -> ()
            }
            frame 8 {
              n4566 = local write "測定新値\nリセット用 9"(w7154) -> ()
            }
            frame 9 {
              n4567 = local write "測定新値\nリセット用 10"(w7155) -> ()
            }
            frame 10 {
            }
            frame 11 {
              n4568 = local write "測定新値\nリセット用 12"(w7156) -> ()
            }
          }
        }
        n4569 = for {
          N: w7132 -> [_]
          tunnel: w7138 -> [w7157]
          i -> [w7158]
          n4570 = case shown="11" w7158 {
            tunnel: w7157 -> [w7159 w7160 w7161 w7162 w7163 w7164 w7165 w7166 w7167 w7168 w7169 w7170]
            frame 0, Default {
              n4571 = property on="メイン測定ボタン_単発 1" class="Bool (指定)"("DisabledEnum"=w7159) -> ()  [unwired: 2 in, 2 out]
              n4572 = property on="メイン測定ボタン_連続 1" class="Bool (指定)"("DisabledEnum"=w7159) -> ()  [unwired: 2 in, 2 out]
            }
            frame 1 {
              n4573 = property on="メイン測定ボタン_単発 2" class="Bool (指定)"("DisabledEnum"=w7160) -> ()  [unwired: 2 in, 2 out]
              n4574 = property on="メイン測定ボタン_連続 2" class="Bool (指定)"("DisabledEnum"=w7160) -> ()  [unwired: 2 in, 2 out]
            }
            frame 2 {
              n4575 = property on="メイン測定ボタン_単発 3" class="Bool (指定)"("DisabledEnum"=w7161) -> ()  [unwired: 2 in, 2 out]
              n4576 = property on="メイン測定ボタン_連続 3" class="Bool (指定)"("DisabledEnum"=w7161) -> ()  [unwired: 2 in, 2 out]
            }
            frame 3 {
              n4577 = property on="メイン測定ボタン_単発 4" class="Bool (指定)"("DisabledEnum"=w7162) -> ()  [unwired: 2 in, 2 out]
              n4578 = property on="メイン測定ボタン_連続 4" class="Bool (指定)"("DisabledEnum"=w7162) -> ()  [unwired: 2 in, 2 out]
            }
            frame 4 {
              n4579 = property on="メイン測定ボタン_単発 5" class="Bool (指定)"("DisabledEnum"=w7163) -> ()  [unwired: 2 in, 2 out]
              n4580 = property on="メイン測定ボタン_連続 5" class="Bool (指定)"("DisabledEnum"=w7163) -> ()  [unwired: 2 in, 2 out]
            }
            frame 5 {
              n4581 = property on="メイン測定ボタン_連続 6" class="Bool (指定)"("DisabledEnum"=w7164) -> ()  [unwired: 2 in, 2 out]
              n4582 = property on="メイン測定ボタン_単発 6" class="Bool (指定)"("DisabledEnum"=w7164) -> ()  [unwired: 2 in, 2 out]
            }
            frame 6 {
              n4583 = property on="メイン測定ボタン_連続 7" class="Bool (指定)"("DisabledEnum"=w7165) -> ()  [unwired: 2 in, 2 out]
              n4584 = property on="メイン測定ボタン_単発 7" class="Bool (指定)"("DisabledEnum"=w7165) -> ()  [unwired: 2 in, 2 out]
            }
            frame 7 {
              n4585 = property on="メイン測定ボタン_単発 8" class="Bool (指定)"("DisabledEnum"=w7166) -> ()  [unwired: 2 in, 2 out]
              n4586 = property on="メイン測定ボタン_連続 8" class="Bool (指定)"("DisabledEnum"=w7166) -> ()  [unwired: 2 in, 2 out]
            }
            frame 8 {
              n4587 = property on="メイン測定ボタン_単発 9" class="Bool (指定)"("DisabledEnum"=w7167) -> ()  [unwired: 2 in, 2 out]
              n4588 = property on="メイン測定ボタン_連続 9" class="Bool (指定)"("DisabledEnum"=w7167) -> ()  [unwired: 2 in, 2 out]
            }
            frame 9 {
              n4589 = property on="メイン測定ボタン_単発 10" class="Bool (指定)"("DisabledEnum"=w7168) -> ()  [unwired: 2 in, 2 out]
              n4590 = property on="メイン測定ボタン_連続 10" class="Bool (指定)"("DisabledEnum"=w7168) -> ()  [unwired: 2 in, 2 out]
            }
            frame 10 {
              n4591 = property on="メイン測定ボタン_単発 11" class="Bool (指定)"("DisabledEnum"=w7169) -> ()  [unwired: 2 in, 2 out]
            }
            frame 11 {
              n4592 = property on="メイン測定ボタン_連続 12" class="Bool (指定)"("DisabledEnum"=w7170) -> ()  [unwired: 2 in, 2 out]
              n4593 = property on="メイン測定ボタン_単発 12" class="Bool (指定)"("DisabledEnum"=w7170) -> ()  [unwired: 2 in, 2 out]
            }
          }
        }
        n4594 = property on="TOPページへ" class="Bool"("DisabledEnum"=w7138) -> ()  [unwired: 2 in, 2 out]
        n4595 = property on="保存して終了" class="Bool"("DisabledEnum"=w7138) -> ()  [unwired: 2 in, 2 out]
        n4596 = property on="保存せずに" class="Bool"("DisabledEnum"=w7138) -> ()  [unwired: 2 in, 2 out]
      }
      event Value Change {
        w7171 = 12
        # "④ボタン操作時の他のボタン操作無効"
        # "※複製時\n①ブールボタン\n測定旧値\nが複製されているか確認\n②測定新値リセット用の作成\n対象の以外をリセットする\n③\nキュー\n④対象の連続ボタン以外複製する"
        # "③"
        # "旧値(ボタンが押される前と後)の値でグローバル_測定キャンセルボタンの\nTrue/Falseの切り替えを行う"
        # "②　例ケースが”メイン測定ボタン_連続2”の場合、\n測定新値リセット用2以外をリセットする"
        # "①"
        n4597 = event-data() -> ("OldVal"=w7172:T6)  [unwired: 1 in, 2 out]
        "測定旧値 12" <- w7172
        n4598 = Enqueue Element(queue=w7181, element="測定12", error in (no error)=w7178) -> (queue out=w7180:refnum<queue>, error out=w7179:errorcluster)  [unwired: 1 in, 1 out]
        n4599 = Select(t=TRUE, s=w7172, f=FALSE) -> (s? t:f=w7175:bool)
        n4600 = global write "測定キャンセルボタン.vi" "グローバル_測定キャンセルボタン"(w7175) -> ()
        n4601 = local write "G_メイン測定キャンセルボタン"(w7175) -> ()
        n4602 = for {
          N: w7171 -> [_]
          tunnel: FALSE -> [w7197]
          i -> [w7198]
          n4603 = case shown="0, デフォルト" w7198 {
            tunnel: w7197 -> [w7199 w7200 w7201 w7202 w7203 w7204 w7205 w7206 w7207 w7208 w7209]
            frame 0, Default {
              n4604 = local write "測定新値\nリセット用 1"(w7199) -> ()
            }
            frame 1 {
              n4605 = local write "測定新値\nリセット用 2"(w7200) -> ()
            }
            frame 2 {
              n4606 = local write "測定新値\nリセット用 3"(w7201) -> ()
            }
            frame 3 {
              n4607 = local write "測定新値\nリセット用 4"(w7202) -> ()
            }
            frame 4 {
              n4608 = local write "測定新値\nリセット用 5"(w7203) -> ()
            }
            frame 5 {
              n4609 = local write "測定新値\nリセット用 6"(w7204) -> ()
            }
            frame 6 {
              n4610 = local write "測定新値\nリセット用 7"(w7205) -> ()
            }
            frame 7 {
              n4611 = local write "測定新値\nリセット用 8"(w7206) -> ()
            }
            frame 8 {
              n4612 = local write "測定新値\nリセット用 9"(w7207) -> ()
            }
            frame 9 {
              n4613 = local write "測定新値\nリセット用 10"(w7208) -> ()
            }
            frame 10 {
              n4614 = local write "測定新値\nリセット用 11"(w7209) -> ()
            }
          }
        }
        n4615 = for {
          N: w7171 -> [_]
          tunnel: w7176 -> [w7183]
          i -> [w7184]
          n4616 = case shown="11" w7184 {
            tunnel: w7183 -> [w7185 w7186 w7187 w7188 w7189 w7190 w7191 w7192 w7193 w7194 w7195 w7196]
            frame 0, Default {
              n4617 = property on="メイン測定ボタン_単発 1" class="Bool (指定)"("DisabledEnum"=w7185) -> ()  [unwired: 2 in, 2 out]
              n4618 = property on="メイン測定ボタン_連続 1" class="Bool (指定)"("DisabledEnum"=w7185) -> ()  [unwired: 2 in, 2 out]
            }
            frame 1 {
              n4619 = property on="メイン測定ボタン_単発 2" class="Bool (指定)"("DisabledEnum"=w7186) -> ()  [unwired: 2 in, 2 out]
              n4620 = property on="メイン測定ボタン_連続 2" class="Bool (指定)"("DisabledEnum"=w7186) -> ()  [unwired: 2 in, 2 out]
            }
            frame 2 {
              n4621 = property on="メイン測定ボタン_単発 3" class="Bool (指定)"("DisabledEnum"=w7187) -> ()  [unwired: 2 in, 2 out]
              n4622 = property on="メイン測定ボタン_連続 3" class="Bool (指定)"("DisabledEnum"=w7187) -> ()  [unwired: 2 in, 2 out]
            }
            frame 3 {
              n4623 = property on="メイン測定ボタン_単発 4" class="Bool (指定)"("DisabledEnum"=w7188) -> ()  [unwired: 2 in, 2 out]
              n4624 = property on="メイン測定ボタン_連続 4" class="Bool (指定)"("DisabledEnum"=w7188) -> ()  [unwired: 2 in, 2 out]
            }
            frame 4 {
              n4625 = property on="メイン測定ボタン_単発 5" class="Bool (指定)"("DisabledEnum"=w7189) -> ()  [unwired: 2 in, 2 out]
              n4626 = property on="メイン測定ボタン_連続 5" class="Bool (指定)"("DisabledEnum"=w7189) -> ()  [unwired: 2 in, 2 out]
            }
            frame 5 {
              n4627 = property on="メイン測定ボタン_連続 6" class="Bool (指定)"("DisabledEnum"=w7190) -> ()  [unwired: 2 in, 2 out]
              n4628 = property on="メイン測定ボタン_単発 6" class="Bool (指定)"("DisabledEnum"=w7190) -> ()  [unwired: 2 in, 2 out]
            }
            frame 6 {
              n4629 = property on="メイン測定ボタン_連続 7" class="Bool (指定)"("DisabledEnum"=w7191) -> ()  [unwired: 2 in, 2 out]
              n4630 = property on="メイン測定ボタン_単発 7" class="Bool (指定)"("DisabledEnum"=w7191) -> ()  [unwired: 2 in, 2 out]
            }
            frame 7 {
              n4631 = property on="メイン測定ボタン_単発 8" class="Bool (指定)"("DisabledEnum"=w7192) -> ()  [unwired: 2 in, 2 out]
              n4632 = property on="メイン測定ボタン_連続 8" class="Bool (指定)"("DisabledEnum"=w7192) -> ()  [unwired: 2 in, 2 out]
            }
            frame 8 {
              n4633 = property on="メイン測定ボタン_単発 9" class="Bool (指定)"("DisabledEnum"=w7193) -> ()  [unwired: 2 in, 2 out]
              n4634 = property on="メイン測定ボタン_連続 9" class="Bool (指定)"("DisabledEnum"=w7193) -> ()  [unwired: 2 in, 2 out]
            }
            frame 9 {
              n4635 = property on="メイン測定ボタン_単発 10" class="Bool (指定)"("DisabledEnum"=w7194) -> ()  [unwired: 2 in, 2 out]
              n4636 = property on="メイン測定ボタン_連続 10" class="Bool (指定)"("DisabledEnum"=w7194) -> ()  [unwired: 2 in, 2 out]
            }
            frame 10 {
              n4637 = property on="メイン測定ボタン_単発 11" class="Bool (指定)"("DisabledEnum"=w7195) -> ()  [unwired: 2 in, 2 out]
              n4638 = property on="メイン測定ボタン_連続 11" class="Bool (指定)"("DisabledEnum"=w7195) -> ()  [unwired: 2 in, 2 out]
            }
            frame 11 {
              n4639 = property on="メイン測定ボタン_単発 12" class="Bool (指定)"("DisabledEnum"=w7196) -> ()  [unwired: 2 in, 2 out]
            }
          }
        }
        n4640 = property on="TOPページへ" class="Bool"("DisabledEnum"=w7176) -> ()  [unwired: 2 in, 2 out]
        n4641 = property on="保存して終了" class="Bool"("DisabledEnum"=w7176) -> ()  [unwired: 2 in, 2 out]
        n4642 = property on="保存せずに" class="Bool"("DisabledEnum"=w7176) -> ()  [unwired: 2 in, 2 out]
      }
      event Value Change {
        w7211 = T8."Disabled" ("無効")
        # "⑤"
        # "※複製時\n①このボタンで操作する以外の\n測定旧値\n測定新値\nを複製して作る\n②ある分だけの\n測定旧値\nを複製して作る\n③ある分だけの\n測定旧値\nを複製して作る\n④はそのまま\n⑤測定新値の\nボタンが複製されているか確認\n⑥Ⅰ.初期設定の\n測定新値_リセットの初期化\nを必ず作る事"
        n4643 = event-data() -> ("NewVal"=w7213:T7)  [unwired: 1 in, 2 out]
        "測定新値 1" <- w7213
        n4644 = local read "書込周期/ms"() -> (w7210:dbl)
        n4645 = Wait (ms)(milliseconds to wait=w7210) -> ()  [unwired: 1 out]
        n4646 = flat-sequence {
          tunnel: w7213 -> [w7240]
          tunnel: w7221 -> [w7241]
          tunnel: w7223 -> [w7242]
          tunnel: [w7242] -> w7217
          tunnel: [w7241] -> w7216
          tunnel: [w7240] -> w7215
          tunnel: [w7239] -> w7214
          tunnel: [w7292] -> w7220
          tunnel: [w7291] -> w7219
          tunnel: [w7290] -> w7218
          tunnel: w7214 -> [w7289]
          tunnel: w7215 -> [w7290]
          tunnel: w7216 -> [w7291]
          tunnel: w7217 -> [w7292]
          tunnel: [w7313] -> w7224
          tunnel: [w7311] -> w7222
          tunnel: w7220 -> [w7312]
          tunnel: w7219 -> [w7310]
          tunnel: w7218 -> [w7309]
          frame #0 {
            w7239 = 32
            # "①測定旧値・新値～32までTrueだったらMAX/MINグローバルリセット"
            n4647 = for {
              N: w7239 -> [_]
              i -> [w7243]
              n4648 = case shown="0, デフォルト" w7243 {
                frame 0, Default {
                }
                frame 1 {
                  n4649 = local read "測定新値\nリセット用 2"() -> (w7244:bool)
                  n4650 = local read "測定旧値 2"() -> (w7245:bool)
                  n4651 = case shown="FALSE" w7244 {
                    frame False {
                    }
                    frame True {
                      n4652 = property on="MAX/MINグローバルリセット用" class="Arr (指定)"() -> ("Value"=w7246:string[][])  [unwired: 2 in, 2 out]
                      n4653 = global write "測定値MAXMIN_G.vi" "測定値MAX/MINグローバル"(w7246) -> ()
                    }
                  }
                  n4654 = case shown="FALSE" w7245 {
                    frame False {
                    }
                    frame True {
                      n4655 = property on="MAX/MINグローバルリセット用" class="Arr (指定)"() -> ("Value"=w7247:string[][])  [unwired: 2 in, 2 out]
                      n4656 = global write "測定値MAXMIN_G.vi" "測定値MAX/MINグローバル"(w7247) -> ()
                    }
                  }
                }
                frame 2 {
                  n4657 = local read "測定新値\nリセット用 3"() -> (w7248:bool)
                  n4658 = local read "測定旧値 3"() -> (w7249:bool)
                  n4659 = case shown="FALSE" w7248 {
                    frame False {
                    }
                    frame True {
                      n4660 = property on="MAX/MINグローバルリセット用" class="Arr (指定)"() -> ("Value"=w7250:string[][])  [unwired: 2 in, 2 out]
                      n4661 = global write "測定値MAXMIN_G.vi" "測定値MAX/MINグローバル"(w7250) -> ()
                    }
                  }
                  n4662 = case shown="FALSE" w7249 {
                    frame False {
                    }
                    frame True {
                      n4663 = property on="MAX/MINグローバルリセット用" class="Arr (指定)"() -> ("Value"=w7251:string[][])  [unwired: 2 in, 2 out]
                      n4664 = global write "測定値MAXMIN_G.vi" "測定値MAX/MINグローバル"(w7251) -> ()
                    }
                  }
                }
                frame 3 {
                  n4665 = local read "測定新値\nリセット用 4"() -> (w7252:bool)
                  n4666 = local read "測定旧値 4"() -> (w7253:bool)
                  n4667 = case shown="FALSE" w7252 {
                    frame False {
                    }
                    frame True {
                      n4668 = property on="MAX/MINグローバルリセット用" class="Arr (指定)"() -> ("Value"=w7254:string[][])  [unwired: 2 in, 2 out]
                      n4669 = global write "測定値MAXMIN_G.vi" "測定値MAX/MINグローバル"(w7254) -> ()
                    }
                  }
                  n4670 = case shown="TRUE" w7253 {
                    frame False {
                    }
                    frame True {
                      n4671 = property on="MAX/MINグローバルリセット用" class="Arr (指定)"() -> ("Value"=w7255:string[][])  [unwired: 2 in, 2 out]
                      n4672 = global write "測定値MAXMIN_G.vi" "測定値MAX/MINグローバル"(w7255) -> ()
                    }
                  }
                }
                frame 4 {
                  n4673 = local read "測定新値\nリセット用 5"() -> (w7256:bool)
                  n4674 = local read "測定旧値 5"() -> (w7257:bool)
                  n4675 = case shown="TRUE" w7256 {
                    frame False {
                    }
                    frame True {
                      n4676 = property on="MAX/MINグローバルリセット用" class="Arr (指定)"() -> ("Value"=w7258:string[][])  [unwired: 2 in, 2 out]
                      n4677 = global write "測定値MAXMIN_G.vi" "測定値MAX/MINグローバル"(w7258) -> ()
                    }
                  }
                  n4678 = case shown="TRUE" w7257 {
                    frame False {
                    }
                    frame True {
                      n4679 = property on="MAX/MINグローバルリセット用" class="Arr (指定)"() -> ("Value"=w7259:string[][])  [unwired: 2 in, 2 out]
                      n4680 = global write "測定値MAXMIN_G.vi" "測定値MAX/MINグローバル"(w7259) -> ()
                    }
                  }
                }
                frame 5 {
                  n4681 = local read "測定新値\nリセット用 6"() -> (w7260:bool)
                  n4682 = local read "測定旧値 6"() -> (w7261:bool)
                  n4683 = case shown="TRUE" w7260 {
                    frame False {
                    }
                    frame True {
                      n4684 = property on="MAX/MINグローバルリセット用" class="Arr (指定)"() -> ("Value"=w7262:string[][])  [unwired: 2 in, 2 out]
                      n4685 = global write "測定値MAXMIN_G.vi" "測定値MAX/MINグローバル"(w7262) -> ()
                    }
                  }
                  n4686 = case shown="TRUE" w7261 {
                    frame False {
                    }
                    frame True {
                      n4687 = property on="MAX/MINグローバルリセット用" class="Arr (指定)"() -> ("Value"=w7263:string[][])  [unwired: 2 in, 2 out]
                      n4688 = global write "測定値MAXMIN_G.vi" "測定値MAX/MINグローバル"(w7263) -> ()
                    }
                  }
                }
                frame 6 {
                  n4689 = local read "測定新値\nリセット用 7"() -> (w7264:bool)
                  n4690 = local read "測定旧値 7"() -> (w7265:bool)
                  n4691 = case shown="TRUE" w7264 {
                    frame False {
                    }
                    frame True {
                      n4692 = property on="MAX/MINグローバルリセット用" class="Arr (指定)"() -> ("Value"=w7266:string[][])  [unwired: 2 in, 2 out]
                      n4693 = global write "測定値MAXMIN_G.vi" "測定値MAX/MINグローバル"(w7266) -> ()
                    }
                  }
                  n4694 = case shown="TRUE" w7265 {
                    frame False {
                    }
                    frame True {
                      n4695 = property on="MAX/MINグローバルリセット用" class="Arr (指定)"() -> ("Value"=w7267:string[][])  [unwired: 2 in, 2 out]
                      n4696 = global write "測定値MAXMIN_G.vi" "測定値MAX/MINグローバル"(w7267) -> ()
                    }
                  }
                }
                frame 7 {
                  n4697 = local read "測定新値\nリセット用 8"() -> (w7268:bool)
                  n4698 = local read "測定旧値 8"() -> (w7269:bool)
                  n4699 = case shown="TRUE" w7268 {
                    frame False {
                    }
                    frame True {
                      n4700 = property on="MAX/MINグローバルリセット用" class="Arr (指定)"() -> ("Value"=w7270:string[][])  [unwired: 2 in, 2 out]
                      n4701 = global write "測定値MAXMIN_G.vi" "測定値MAX/MINグローバル"(w7270) -> ()
                    }
                  }
                  n4702 = case shown="TRUE" w7269 {
                    frame False {
                    }
                    frame True {
                      n4703 = property on="MAX/MINグローバルリセット用" class="Arr (指定)"() -> ("Value"=w7271:string[][])  [unwired: 2 in, 2 out]
                      n4704 = global write "測定値MAXMIN_G.vi" "測定値MAX/MINグローバル"(w7271) -> ()
                    }
                  }
                }
                frame 8 {
                  n4705 = local read "測定新値\nリセット用 9"() -> (w7272:bool)
                  n4706 = local read "測定旧値 9"() -> (w7273:bool)
                  n4707 = case shown="TRUE" w7272 {
                    frame False {
                    }
                    frame True {
                      n4708 = property on="MAX/MINグローバルリセット用" class="Arr (指定)"() -> ("Value"=w7274:string[][])  [unwired: 2 in, 2 out]
                      n4709 = global write "測定値MAXMIN_G.vi" "測定値MAX/MINグローバル"(w7274) -> ()
                    }
                  }
                  n4710 = case shown="TRUE" w7273 {
                    frame False {
                    }
                    frame True {
                      n4711 = property on="MAX/MINグローバルリセット用" class="Arr (指定)"() -> ("Value"=w7275:string[][])  [unwired: 2 in, 2 out]
                      n4712 = global write "測定値MAXMIN_G.vi" "測定値MAX/MINグローバル"(w7275) -> ()
                    }
                  }
                }
                frame 9 {
                  n4713 = local read "測定新値\nリセット用 10"() -> (w7276:bool)
                  n4714 = local read "測定旧値 10"() -> (w7277:bool)
                  n4715 = case shown="TRUE" w7276 {
                    frame False {
                    }
                    frame True {
                      n4716 = property on="MAX/MINグローバルリセット用" class="Arr (指定)"() -> ("Value"=w7278:string[][])  [unwired: 2 in, 2 out]
                      n4717 = global write "測定値MAXMIN_G.vi" "測定値MAX/MINグローバル"(w7278) -> ()
                    }
                  }
                  n4718 = case shown="TRUE" w7277 {
                    frame False {
                    }
                    frame True {
                      n4719 = property on="MAX/MINグローバルリセット用" class="Arr (指定)"() -> ("Value"=w7279:string[][])  [unwired: 2 in, 2 out]
                      n4720 = global write "測定値MAXMIN_G.vi" "測定値MAX/MINグローバル"(w7279) -> ()
                    }
                  }
                }
                frame 10 {
                  n4721 = local read "測定新値\nリセット用 11"() -> (w7280:bool)
                  n4722 = local read "測定旧値 11"() -> (w7281:bool)
                  n4723 = case shown="TRUE" w7280 {
                    frame False {
                    }
                    frame True {
                      n4724 = property on="MAX/MINグローバルリセット用" class="Arr (指定)"() -> ("Value"=w7282:string[][])  [unwired: 2 in, 2 out]
                      n4725 = global write "測定値MAXMIN_G.vi" "測定値MAX/MINグローバル"(w7282) -> ()
                    }
                  }
                  n4726 = case shown="TRUE" w7281 {
                    frame False {
                    }
                    frame True {
                      n4727 = property on="MAX/MINグローバルリセット用" class="Arr (指定)"() -> ("Value"=w7283:string[][])  [unwired: 2 in, 2 out]
                      n4728 = global write "測定値MAXMIN_G.vi" "測定値MAX/MINグローバル"(w7283) -> ()
                    }
                  }
                }
                frame 11 {
                  n4729 = local read "測定新値\nリセット用 12"() -> (w7284:bool)
                  n4730 = local read "測定旧値 12"() -> (w7285:bool)
                  n4731 = case shown="TRUE" w7284 {
                    frame False {
                    }
                    frame True {
                      n4732 = property on="MAX/MINグローバルリセット用" class="Arr (指定)"() -> ("Value"=w7286:string[][])  [unwired: 2 in, 2 out]
                      n4733 = global write "測定値MAXMIN_G.vi" "測定値MAX/MINグローバル"(w7286) -> ()
                    }
                  }
                  n4734 = case shown="TRUE" w7285 {
                    frame False {
                    }
                    frame True {
                      n4735 = property on="MAX/MINグローバルリセット用" class="Arr (指定)"() -> ("Value"=w7287:string[][])  [unwired: 2 in, 2 out]
                      n4736 = global write "測定値MAXMIN_G.vi" "測定値MAX/MINグローバル"(w7287) -> ()
                    }
                  }
                }
              }
            }
          }
          frame #1 {
            w7288 = FALSE
            # "②測定新規リセット用、測定旧値のリセット"
            n4737 = global write "測定キャンセルボタン.vi" "グローバル_測定キャンセルボタン"(w7288) -> ()
            n4738 = local write "G_メイン測定キャンセルボタン"(w7288) -> ()
            n4739 = for {
              N: w7289 -> [_]
              tunnel: w7288 -> [w7293]
              i -> [w7294]
              n4740 = case shown="0, デフォルト" w7294 {
                tunnel: w7293 -> [w7295 w7296 w7297 w7298 w7299 w7300 w7301 w7302 w7303 w7304 w7305 w7306]
                frame 0, Default {
                  n4741 = local write "測定新値\nリセット用 1"(w7295) -> ()
                  n4742 = local write "測定旧値 1"(w7295) -> ()
                }
                frame 1 {
                  n4743 = local write "測定新値\nリセット用 2"(w7296) -> ()
                  n4744 = local write "測定旧値 2"(w7296) -> ()
                }
                frame 2 {
                  n4745 = local write "測定新値\nリセット用 3"(w7297) -> ()
                  n4746 = local write "測定旧値 3"(w7297) -> ()
                }
                frame 3 {
                  n4747 = local write "測定新値\nリセット用 4"(w7298) -> ()
                  n4748 = local write "測定旧値 4"(w7298) -> ()
                }
                frame 4 {
                  n4749 = local write "測定新値\nリセット用 5"(w7299) -> ()
                  n4750 = local write "測定旧値 5"(w7299) -> ()
                }
                frame 5 {
                  n4751 = local write "測定新値\nリセット用 6"(w7300) -> ()
                  n4752 = local write "測定旧値 6"(w7300) -> ()
                }
                frame 6 {
                  n4753 = local write "測定新値\nリセット用 7"(w7301) -> ()
                  n4754 = local write "測定旧値 7"(w7301) -> ()
                }
                frame 7 {
                  n4755 = local write "測定新値\nリセット用 8"(w7302) -> ()
                  n4756 = local write "測定旧値 8"(w7302) -> ()
                }
